vi "VI Server Control N2 Text Out.vi"(1 "VI Server Control N2":T2={"VI name"="", "Control"=[], "Value"=[], "Boolean?"=[], "Wait Option"=enum."Wait Until", "wait (sec)"=10.0, "Control to End"="", "finish boolean?"=enum."boolean", "Condition"=enum."<= target value", "Target Value"=0.0, "xxx%"=0.0, "update every (s)"=120.0, "Timeout (sec)"=10000.0} {"Boolean?" min=0.0 max=1.0 step=1.0 format="%#_1g"}) -> (0 "Command text":string[][](array[string]))   [LabVIEW 2020]
uses:
  VI Server Control N2.ctl
  condition.ctl
panel:
  out "Wait Option":enum32{"Wait Until", "Do Not Wait"}(ring)
  out "Condition":T1
  out "finish boolean?":enum32{"boolean", "not boolean"}(ring)
  out "Long Description":string
  out "Est Time (H:M:S)":dbl
  out "String Cluster":T3
  # "Value of Control\n(if control is boolean type\n1 for \"ON\" and,0 for \"OFF\")"
  # "Is this control Boolean?\n(Yes: 1,  No: 0)"
  # "Name of  Control"
  # "0"
  # "1"
  # "2"
  # "3"
  # "4"
  # "5"
  # "6"
  # "7"
  # "8"
  # "9"
  # "1."
  # "Purely wait for"
  # "seconds"
  # "2."
  # "Control / Indicator Name"
  # "which is"
  # "Finish if"
  # "meets the following conditions"
  # "(check and update every"
  # "seconds)"
  # "3. Timeout"
  # "Wait until the following condition meets."
  # "Do not wait and move on to the next line in sequence."
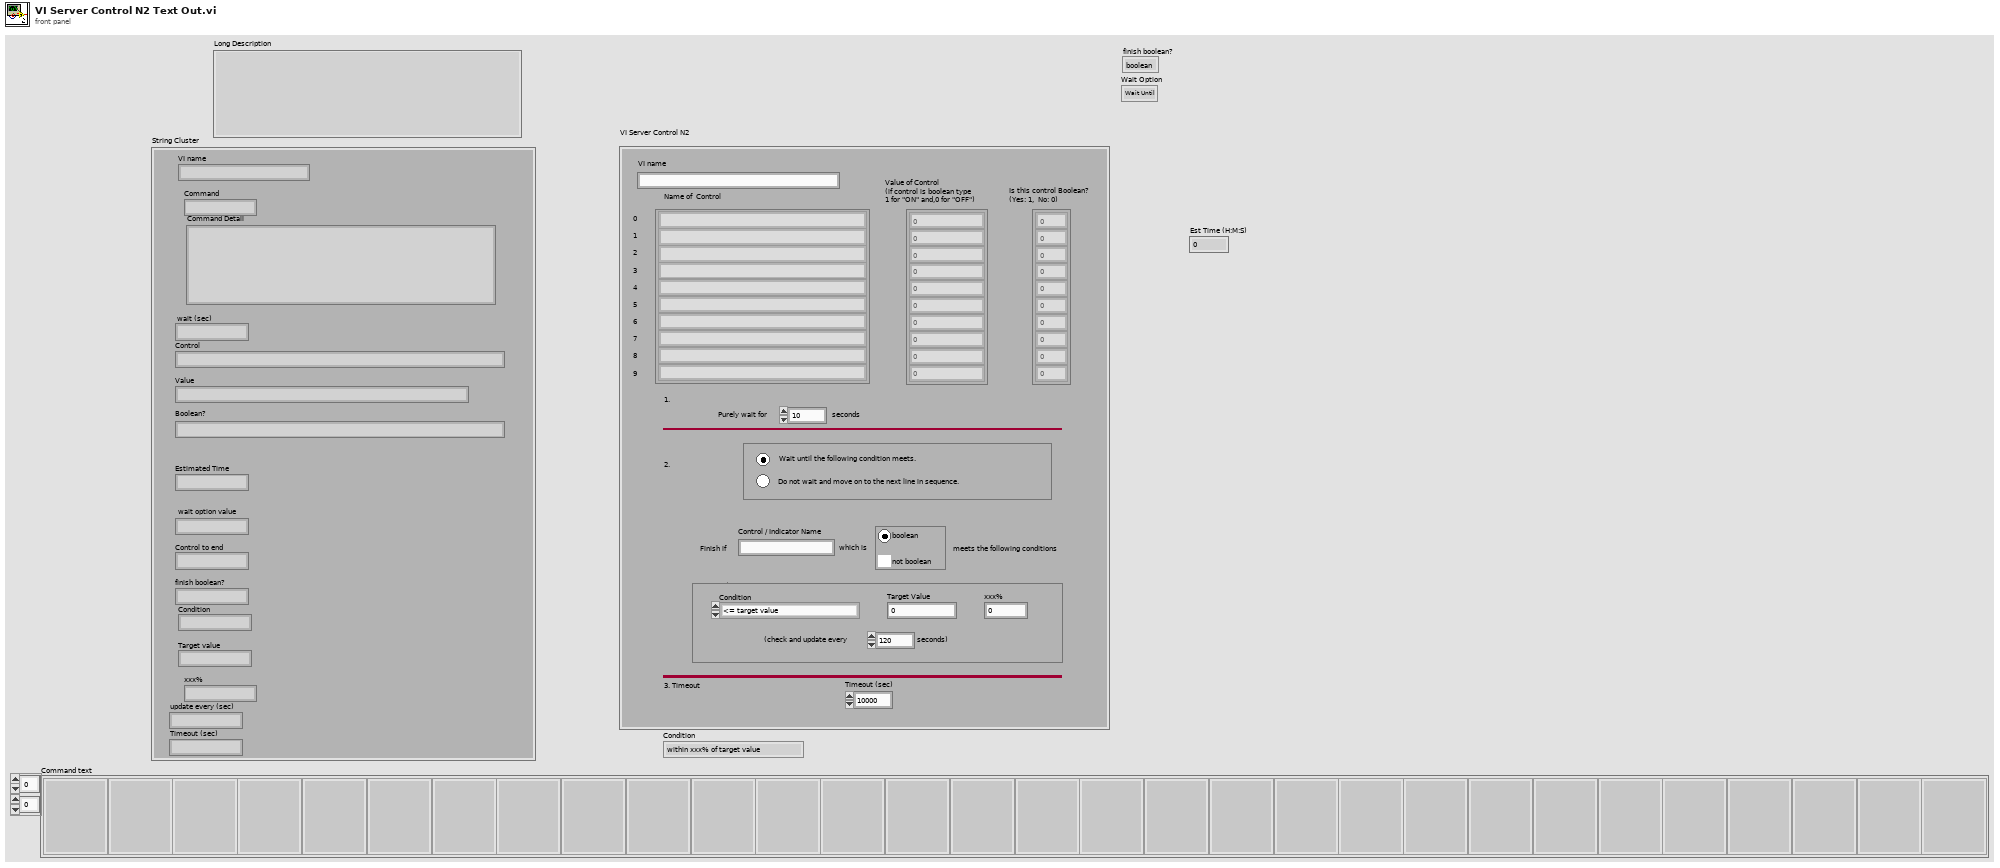
[diagram p1: front panel]
types:
  T1 = typedef "condition.ctl" = enum16{"within xxx% of target value", "<= target value", ">= target value", "= target value", "Boolean ON", "Boolean OFF"}
  T2 = typedef "VI Server Control N2.ctl" = cluster{"VI name":string, "Control":string[], "Value":dbl[], "Boolean?":dbl[], "Wait Option":enum32{"Wait Until", "Do Not Wait"}, "wait (sec)":dbl, "Control to End":string, "finish boolean?":enum32{"boolean", "not boolean"}, "Condition":T1, "Target Value":dbl, "xxx%":dbl, "update every (s)":dbl, "Timeout (sec)":dbl}
  T3 = cluster{"VI name":string, "Command":string, "Command Detail":string, " wait (sec)":string, "Control":string, "Value":string, "Estimated Time":string, "Boolean?":string, "wait option value":string, "Control to end":string, "finish boolean?":string, "Condition":string, "Target value":string, "xxx%":string, "update every (sec)":string, "Timeout (sec)":string}
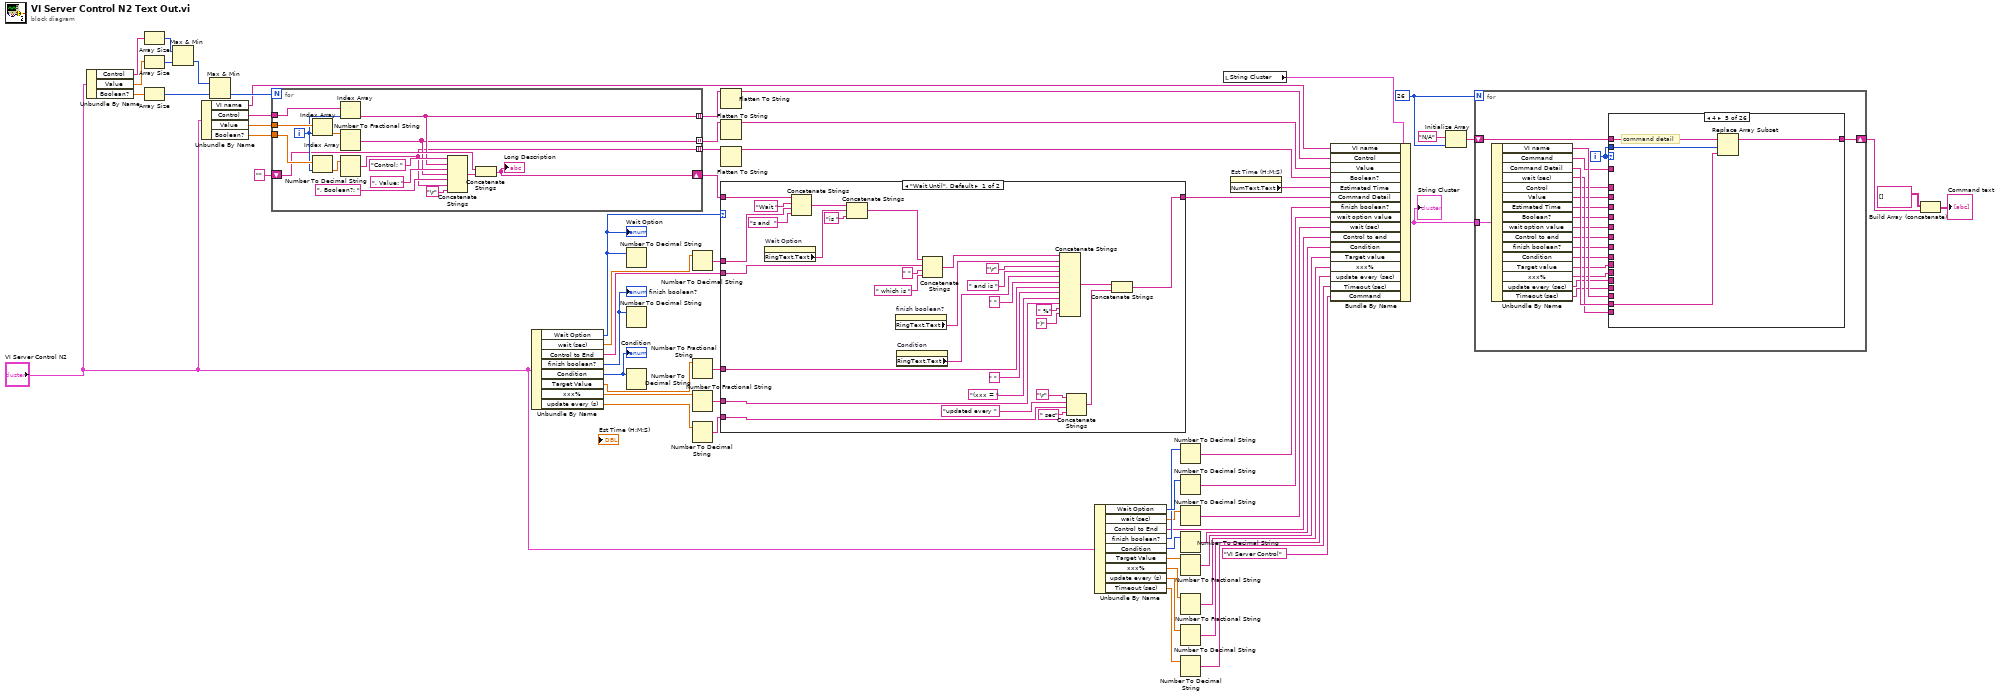
[diagram p0: block diagram]
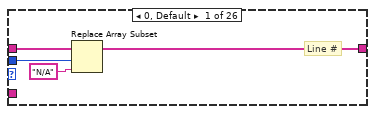
[diagram p3: hidden frame]
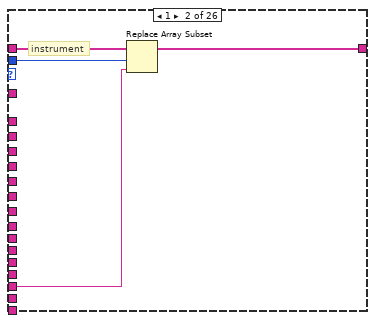
[diagram p4: hidden frame]
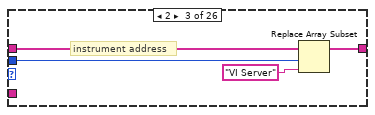
[diagram p5: hidden frame]
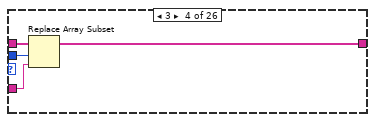
[diagram p6: hidden frame]
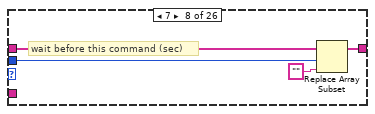
[diagram p9: hidden frame]
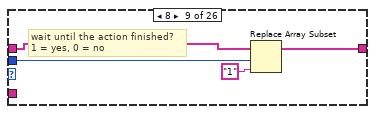
[diagram p10: hidden frame]
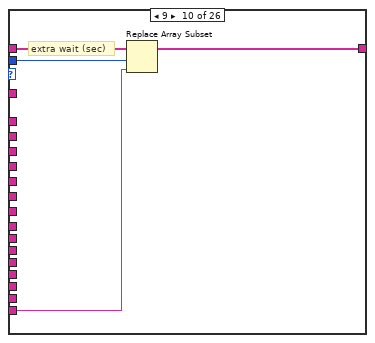
[diagram p11: hidden frame]
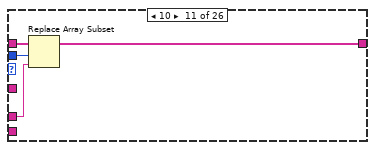
[diagram p12: hidden frame]
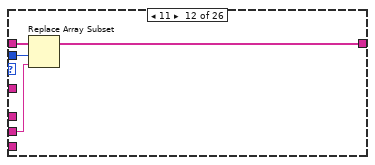
[diagram p13: hidden frame]
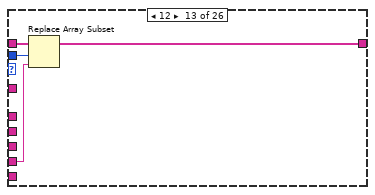
[diagram p14: hidden frame]
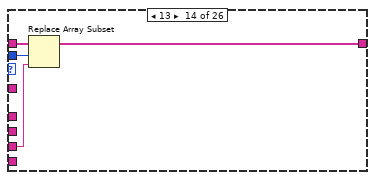
[diagram p15: hidden frame]
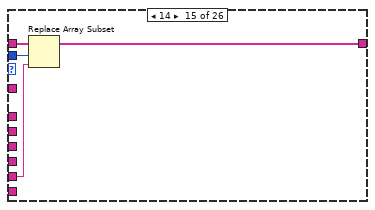
[diagram p16: hidden frame]
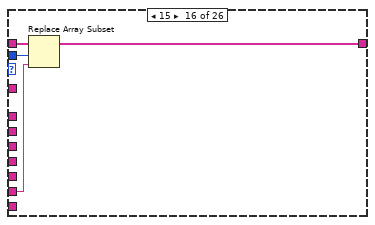
[diagram p17: hidden frame]
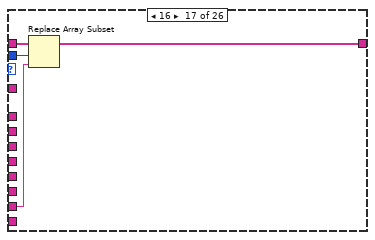
[diagram p18: hidden frame]
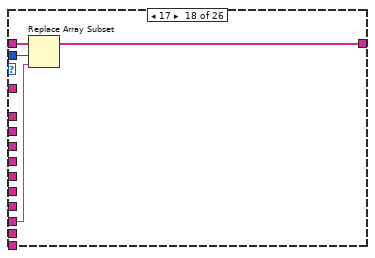
[diagram p19: hidden frame]
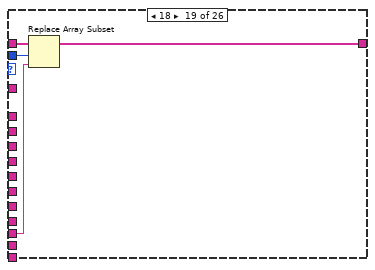
[diagram p20: hidden frame]
diagram:
  w59 = 26
  n1 = Unbundle By Name("VI Server Control N2") -> ("Control"=w54:string[], "Value"=w52:dbl[], "Boolean?"=w50:dbl[])
  n2 = Array Size(array=w54) -> (size(s)=w53:i32)
  n3 = Array Size(array=w52) -> (size(s)=w51:i32)
  n4 = Array Size(array=w50) -> (size(s)=w49:i32)
  n5 = Max & Min(x=w53, y=w51) -> (min(x,y)=w48:i32)  [unwired: 1 out]
  n6 = Unbundle By Name("VI Server Control N2") -> ("VI name"=w40:string, "Control"=w46:string[], "Value"=w45:dbl[], "Boolean?"=w44:dbl[])
  n7 = Max & Min(x=w48, y=w49) -> (min(x,y)=w47:i32)  [unwired: 1 out]
  n8 = for {
    N: w47 -> [_]
    tunnel: w46 -> [w77]
    tunnel: w45 -> [w76]
    tunnel: w44 -> [w75]
    shift-right: [w65] -> w36
    shift-left: "" -> [w67]
    tunnel: [w64] -> w43 mode=indexing
    tunnel: [w63] -> w42 mode=indexing
    tunnel: [w62] -> w41 mode=indexing
    i -> [w74]
    n9 = Index Array(array=w76, index=w74) -> (element=w72:dbl)
    n10 = Index Array(array=w75, index=w74) -> (element=w73:dbl)
    n11 = Index Array(array=w77, index=w74) -> (element=w64:string)
    n12 = Number To Fractional String(number=w72) -> (F-format string=w63:string)  [unwired: 3 in]
    n13 = Number To Decimal String(number=w73) -> (decimal integer string=w62:string)  [unwired: 1 in]
    n14 = Concatenate Strings("Control: " ("string"), w64, ", Value: " ("string"), w63, ", Boolean?: " ("string"), w62, "\r") -> (w66:string)
    n15 = Concatenate Strings(w67, w66) -> (w65:string)
    "Long Description" <- w65
  }
  n16 = Unbundle By Name("VI Server Control N2") -> ("Wait Option"=w25:enum32{"Wait Until", "Do Not Wait"}, "wait (sec)"=w35:dbl, "Control to End"=w33:string, "finish boolean?"=w24:enum32{"boolean", "not boolean"}, "Condition"=w23:T1, "Target Value"=w32:dbl, "xxx%"=w30:dbl, "update every (s)"=w28:dbl)
  "finish boolean?" <- w24
  "Condition" <- w23
  "Wait Option" <- w25
  n17 = Number To Decimal String(number=w25) -> ()  [unwired: 1 in, 1 out]
  n18 = Number To Decimal String(number=w24) -> ()  [unwired: 1 in, 1 out]
  n19 = Number To Decimal String(number=w23) -> ()  [unwired: 1 in, 1 out]
  n20 = Number To Decimal String(number=w35) -> (decimal integer string=w34:string)  [unwired: 1 in]
  n21 = Number To Fractional String(number=w32) -> (F-format string=w31:string)  [unwired: 3 in]
  n22 = Number To Fractional String(number=w30) -> (F-format string=w29:string)  [unwired: 3 in]
  n23 = Number To Decimal String(number=w28) -> (decimal integer string=w27:string)  [unwired: 1 in]
  n24 = Flatten To String(anything=w43) -> (data string=w3:string)  [unwired: 3 in, 2 out]
  n25 = Flatten To String(anything=w42) -> (data string=w39:string)  [unwired: 3 in, 2 out]
  n26 = Flatten To String(anything=w41) -> (data string=w38:string)  [unwired: 3 in, 2 out]
  n27 = case shown="\"Wait Until\", Default" w25 {
    tunnel: w36 -> [w103 w108]
    tunnel: w34 -> [w100 _]
    tunnel: w33 -> [w98 _]
    tunnel: w31 -> [w93 _]
    tunnel: w29 -> [w91 _]
    tunnel: w27 -> [w88 _]
    tunnel: [w84 w108] -> w26
    frame "Wait Until", Default {
      n28 = property on="Wait Option" class="Enum (strict)"() -> ("RingText.Text"=w107:string)  [unwired: 2 in, 2 out]
      n29 = Concatenate Strings(w103, "Wait " ("string"), w100, "s and  " ("string")) -> (w102:string)
      n30 = Concatenate Strings(w102, w107, "is " ("string")) -> (w105:string)
      n31 = property on="finish boolean?" class="Enum (strict)"() -> ("RingText.Text"=w96:string)  [unwired: 2 in, 2 out]
      n32 = property on="Condition" class="Enum (strict)"() -> ("RingText.Text"=w94:string)  [unwired: 2 in, 2 out]
      n33 = Concatenate Strings(w105, w98, " " ("string"), " which is " ("string")) -> (w97:string)
      n34 = Concatenate Strings(w97, w96, "\r", " and is " ("string"), w94, " " ("string"), w93, " " ("string"), "(xxx = " ("string"), w91, " %" ("string"), ")" ("string")) -> (w86:string)
      n35 = Concatenate Strings("\r", "updated every " ("string"), w88, " sec" ("string")) -> (w85:string)
      n36 = Concatenate Strings(w86, w85) -> (w84:string)
    }
    frame "Do Not Wait" {
    }
  }
  n37 = Unbundle By Name("VI Server Control N2") -> ("Wait Option"=w22:enum32{"Wait Until", "Do Not Wait"}, "wait (sec)"=w18:dbl, "Control to End"=w14:string, "finish boolean?"=w21:enum32{"boolean", "not boolean"}, "Condition"=w20:T1, "Target Value"=w12:dbl, "xxx%"=w10:dbl, "update every (s)"=w8:dbl, "Timeout (sec)"=w6:dbl)
  n38 = Number To Decimal String(number=w21) -> (decimal integer string=w16:string)  [unwired: 1 in]
  n39 = Number To Decimal String(number=w22) -> (decimal integer string=w17:string)  [unwired: 1 in]
  n40 = Number To Decimal String(number=w18) -> (decimal integer string=w15:string)  [unwired: 1 in]
  n41 = Number To Decimal String(number=w20) -> (decimal integer string=w13:string)  [unwired: 1 in]
  n42 = Number To Fractional String(number=w12) -> (F-format string=w11:string)  [unwired: 3 in]
  n43 = Number To Fractional String(number=w10) -> (F-format string=w9:string)  [unwired: 3 in]
  n44 = Number To Decimal String(number=w8) -> (decimal integer string=w7:string)  [unwired: 1 in]
  n45 = Number To Decimal String(number=w6) -> (decimal integer string=w5:string)  [unwired: 1 in]
  n46 = local read "String Cluster"() -> (w56:T3)
  n47 = property on="Est Time (H:M:S)" class="DigNum (strict)"() -> ("NumText.Text"=w37:string)  [unwired: 2 in, 2 out]
  n48 = Bundle By Name(cluster=w56, "VI name"=w40, "Control"=w3, "Value"=w39, "Boolean?"=w38, "Estimated Time"=w37, "Command Detail"=w26, "finish boolean?"=w16, "wait option value"=w17, "wait (sec)"=w15, "Control to end"=w14, "Condition"=w13, "Target value"=w11, "xxx%"=w9, "update every (sec)"=w7, "Timeout (sec)"=w5, "Command"="VI Server Control") -> (w55:T3)
  "String Cluster" <- w55
  n49 = Initialize Array("N/A", w59) -> (w58:string[])
  n50 = for {
    N: w59 -> [_]
    shift-right: [w126] -> w57
    shift-left: w58 -> [w127]
    tunnel: w55 -> [w125]
    i -> [w128]
    n51 = Unbundle By Name(w125) -> ("VI name"=w124:string, "Command"=w123:string, "Command Detail"=w122:string, "wait (sec)"=w121:string, "Control"=w120:string, "Value"=w119:string, "Estimated Time"=w117:string, "Boolean?"=w118:string, "wait option value"=w116:string, "Control to end"=w115:string, "finish boolean?"=w114:string, "Condition"=w113:string, "Target value"=w112:string, "xxx%"=w111:string, "update every (sec)"=w110:string, "Timeout (sec)"=w109:string)
    n52 = case shown="4" w128 {
      tunnel: w128 -> [w131 w136 w140 w143 w147 _ _ w152 w156 w160 w166 w168 w172 w177 w180 w184 w188 w192 w196 w200 w204 w208 _ _ _ _]
      tunnel: w127 -> [w132 w135 w139 w144 w148 w149 w150 w154 w158 w162 w164 w169 w174 w178 w182 w186 w190 w194 w198 w202 w206 w210 w211 w212 w213 w214]
      tunnel: [w129 w134 w138 w142 w146 w149 w150 w153 w157 w161 w163 w170 w173 w175 w181 w185 w189 w193 w197 w201 w205 w209 w211 w212 w213 w214] -> w126
      tunnel: w124 -> [_ w133 _ _ _ _ _ _ _ _ _ _ _ _ _ _ _ _ _ _ _ _ _ _ _ _]
      tunnel: w123 -> [_ _ _ w141 _ _ _ _ _ _ _ _ _ _ _ _ _ _ _ _ _ _ _ _ _ _]
      tunnel: w122 -> [_ _ _ _ w145 _ _ _ _ _ _ _ _ _ _ _ _ _ _ _ _ _ _ _ _ _]
      tunnel: w121 -> [_ _ _ _ _ _ _ _ _ w159 _ _ _ _ _ _ _ _ _ _ _ _ _ _ _ _]
      tunnel: w120 -> [_ _ _ _ _ _ _ _ _ _ w165 _ _ _ _ _ _ _ _ _ _ _ _ _ _ _]
      tunnel: w119 -> [_ _ _ _ _ _ _ _ _ _ _ w167 _ _ _ _ _ _ _ _ _ _ _ _ _ _]
      tunnel: w118 -> [_ _ _ _ _ _ _ _ _ _ _ _ w171 _ _ _ _ _ _ _ _ _ _ _ _ _]
      tunnel: w117 -> [_ _ _ _ _ _ _ _ _ _ _ _ _ w176 _ _ _ _ _ _ _ _ _ _ _ _]
      tunnel: w116 -> [_ _ _ _ _ _ _ _ _ _ _ _ _ _ w179 _ _ _ _ _ _ _ _ _ _ _]
      tunnel: w115 -> [_ _ _ _ _ _ _ _ _ _ _ _ _ _ _ w183 _ _ _ _ _ _ _ _ _ _]
      tunnel: w114 -> [_ _ _ _ _ _ _ _ _ _ _ _ _ _ _ _ w187 _ _ _ _ _ _ _ _ _]
      tunnel: w113 -> [_ _ _ _ _ _ _ _ _ _ _ _ _ _ _ _ _ w191 _ _ _ _ _ _ _ _]
      tunnel: w112 -> [_ _ _ _ _ _ _ _ _ _ _ _ _ _ _ _ _ _ w195 _ _ _ _ _ _ _]
      tunnel: w111 -> [_ _ _ _ _ _ _ _ _ _ _ _ _ _ _ _ _ _ _ w199 _ _ _ _ _ _]
      tunnel: w110 -> [_ _ _ _ _ _ _ _ _ _ _ _ _ _ _ _ _ _ _ _ w203 _ _ _ _ _]
      tunnel: w109 -> [_ _ _ _ _ _ _ _ _ _ _ _ _ _ _ _ _ _ _ _ _ w207 _ _ _ _]
      frame 0, Default {
        # "Line #"
        n53 = Replace Array Subset(array=w132, new element="N/A", index=w131) -> (w129:string[])
      }
      frame 1 {
        # "instrument"
        n54 = Replace Array Subset(array=w135, new element=w133, index=w136) -> (w134:string[])
      }
      frame 2 {
        # "instrument address"
        n55 = Replace Array Subset(array=w139, new element="VI Server" ("new element/subarray"), index=w140) -> (w138:string[])
      }
      frame 3 {
        n56 = Replace Array Subset(array=w144, new element=w141, index=w143) -> (w142:string[])
      }
      frame 4 {
        # "command detail"
        n57 = Replace Array Subset(array=w148, new element=w145, index=w147) -> (w146:string[])
      }
      frame 5 {
        # "in  case 1"
      }
      frame 6 {
        # "in case 2"
      }
      frame 7 {
        # "wait before this command (sec)"
        n58 = Replace Array Subset(array=w154, new element="" ("new element/subarray"), index=w152) -> (w153:string[])
      }
      frame 8 {
        # "wait until the action finished?\n1 = yes, 0 = no"
        n59 = Replace Array Subset(array=w158, new element="1", index=w156) -> (w157:string[])
      }
      frame 9 {
        # "extra wait (sec)"
        n60 = Replace Array Subset(array=w162, new element=w159, index=w160) -> (w161:string[])
      }
      frame 10 {
        n61 = Replace Array Subset(array=w164, new element=w165, index=w166) -> (w163:string[])
      }
      frame 11 {
        n62 = Replace Array Subset(array=w169, new element=w167, index=w168) -> (w170:string[])
      }
      frame 12 {
        n63 = Replace Array Subset(array=w174, new element=w171, index=w172) -> (w173:string[])
      }
      frame 13 {
        n64 = Replace Array Subset(array=w178, new element=w176, index=w177) -> (w175:string[])
      }
      frame 14 {
        n65 = Replace Array Subset(array=w182, new element=w179, index=w180) -> (w181:string[])
      }
      frame 15 {
        n66 = Replace Array Subset(array=w186, new element=w183, index=w184) -> (w185:string[])
      }
      frame 16 {
        n67 = Replace Array Subset(array=w190, new element=w187, index=w188) -> (w189:string[])
      }
      frame 17 {
        n68 = Replace Array Subset(array=w194, new element=w191, index=w192) -> (w193:string[])
      }
      frame 18 {
        n69 = Replace Array Subset(array=w198, new element=w195, index=w196) -> (w197:string[])
      }
      frame 19 {
        n70 = Replace Array Subset(array=w202, new element=w199, index=w200) -> (w201:string[])
      }
      frame 20 {
        n71 = Replace Array Subset(array=w206, new element=w203, index=w204) -> (w205:string[])
      }
      frame 21 {
        n72 = Replace Array Subset(array=w210, new element=w207, index=w208) -> (w209:string[])
      }
      frame 22 {
      }
      frame 23 {
      }
      frame 24 {
      }
      frame 25 {
      }
    }
  }
  n73 = Build Array (concatenate)(string[][] [], w57) -> (→"Command text":string[][])
